vi "关键参数区转CDAB.vi"(11 "关键参数区":T1) -> (3 "输出数组":u16[](array[numeric]))   [LabVIEW 2016]
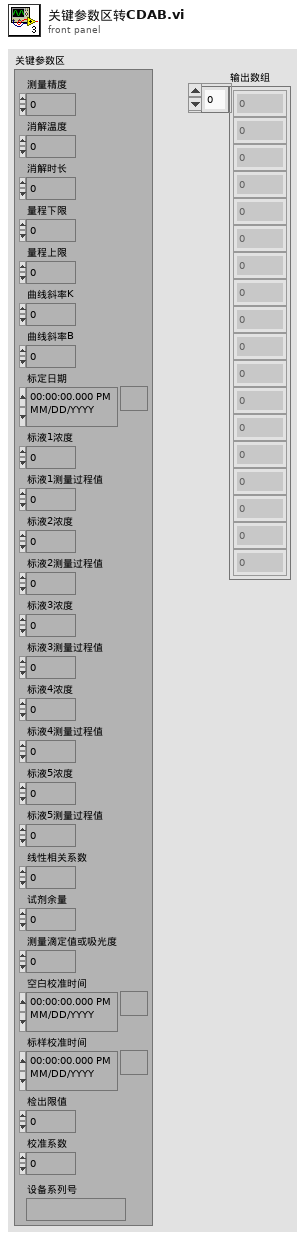
[diagram p1: front panel]
types:
  T1 = cluster{"测量精度":u16, "消解温度":u16, "消解时长":u16, "量程下限":sgl, "量程上限":sgl, "曲线斜率K":sgl, "曲线斜率B":sgl, "标定日期":timestamp, "标液1浓度":sgl, "标液1测量过程值":sgl, "标液2浓度":sgl, "标液2测量过程值":sgl, "标液3浓度":sgl, "标液3测量过程值":sgl, "标液4浓度":sgl, "标液4测量过程值":sgl, "标液5浓度":sgl, "标液5测量过程值":sgl, "线性相关系数":sgl, "试剂余量":u32, "测量滴定值或吸光度":sgl, "空白校准时间":timestamp, "标样校准时间":timestamp, "检出限值":sgl, "校准系数":sgl, "设备系列号":string}
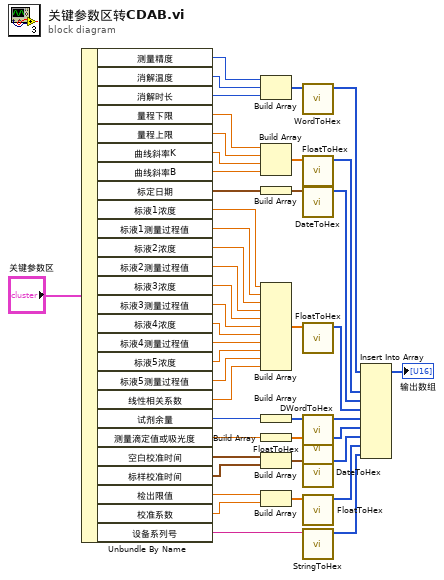
[diagram p0: block diagram]
diagram:
  n1 = Unbundle By Name("关键参数区") -> ("测量精度"=w43:u16, "消解温度"=w42:u16, "消解时长"=w41:u16, "量程下限"=w40:sgl, "量程上限"=w39:sgl, "曲线斜率K"=w38:sgl, "曲线斜率B"=w37:sgl, "标定日期"=w34:timestamp, "标液1浓度"=w32:sgl, "标液1测量过程值"=w31:sgl, "标液2浓度"=w30:sgl, "标液2测量过程值"=w29:sgl, "标液3浓度"=w28:sgl, "标液3测量过程值"=w27:sgl, "标液4浓度"=w26:sgl, "标液4测量过程值"=w25:sgl, "标液5浓度"=w24:sgl, "标液5测量过程值"=w23:sgl, "线性相关系数"=w22:sgl, "试剂余量"=w21:u32, "测量滴定值或吸光度"=w19:sgl, "空白校准时间"=w17:timestamp, "标样校准时间"=w15:timestamp, "检出限值"=w14:sgl, "校准系数"=w13:sgl, "设备系列号"=w11:string)
  n2 = Build Array(w43, w42, w41) -> (w44:u16[])
  n3 = Build Array(w40, w39, w38, w37) -> (w36:sgl[])
  n4 = Build Array(w34) -> (w35:timestamp[])
  n5 = Build Array(w32, w31, w30, w29, w28, w27, w26, w25, w24, w23, w22) -> (w33:sgl[])
  n6 = Build Array(w21) -> (w20:u32[])
  n7 = Build Array(w19) -> (w18:sgl[])
  n8 = Build Array(w17, w15) -> (w16:timestamp[])
  n9 = Build Array(w14, w13) -> (w12:sgl[])
  n10 = call "WordToHex.vi"("WORD"=w44) -> ("数组"=w10:u16[])  [unwired: 10 in]
  n11 = call "FloatToHex.vi"("浮点数"=w36) -> ("DCBA整形输出"=w9:u16[])  [unwired: 10 in]
  n12 = call "DateToHex.vi"("DATE"=w35) -> ("数组"=w8:u16[])  [unwired: 10 in]
  n13 = call "FloatToHex.vi"("浮点数"=w33) -> ("DCBA整形输出"=w7:u16[])  [unwired: 10 in]
  n14 = call "DWordToHex.vi"("DWORD"=w20) -> ("数组"=w6:u16[])  [unwired: 10 in]
  n15 = call "FloatToHex.vi"("浮点数"=w18) -> ("DCBA整形输出"=w5:u16[])  [unwired: 10 in]
  n16 = call "DateToHex.vi"("DATE"=w16) -> ("数组"=w4:u16[])  [unwired: 10 in]
  n17 = call "FloatToHex.vi"("浮点数"=w12) -> ("DCBA整形输出"=w3:u16[])  [unwired: 10 in]
  n18 = call "StringToHex.vi"("字符串"=w11) -> ("数组"=w2:u16[])  [unwired: 10 in]
  n19 = Insert Into Array(array=w10, new element #1=w9, new element #2=w8, new element #3=w7, new element #4=w6, new element #5=w5, new element #6=w4, new element #7=w3, new element #8=w2) -> (→"输出数组":u16[])  [unwired: 1 in]
